vi "Coord window-PictureMap abs max.vi"(11 "Coordinates Listbox Item Names":string[][](array[string])) -> (1 "Auto-scale":bool, 3 "Absolute maximum coordinate (inc current position)":dbl)   [LabVIEW 2013]
panel:
  out "Absolute maximum coordinate in the list":dbl
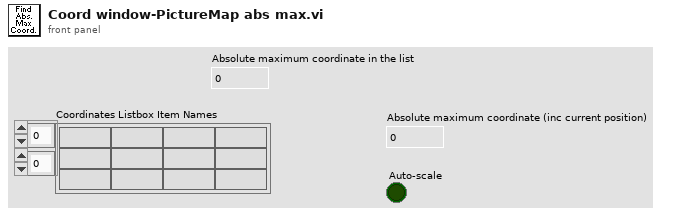
[diagram p1: front panel]
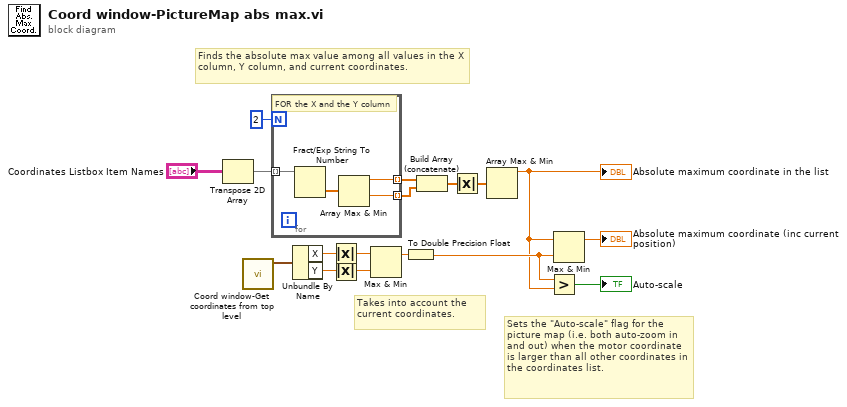
[diagram p0: block diagram]
diagram:
  # "Sets the \"Auto-scale\" flag for the picture map (i.e. both auto-zoom in and out) when the motor coordinate is larger than all other coordinates in the coordinates list."
  # "Takes into account the current coordinates."
  # "Finds the absolute max value among all values in the X column, Y column, and current coordinates."
  n1 = Transpose 2D Array(2D array="Coordinates Listbox Item Names") -> (transposed array=w13:string[][])
  n2 = call "Coord window-Get coordinates from top level.vi"() -> ("Coordinates"=w10:cluster{"X":sgl, "Y":sgl, "Z":sgl})  [unwired: 11 in]
  n3 = for {
    N: 2 -> [_]
    tunnel: w13 -> [w21] mode=indexing
    tunnel: [w19] -> w14 mode=indexing
    tunnel: [w18] -> w15 mode=indexing
    # "FOR the X and the Y column"
    n4 = Fract/Exp String To Number(string=w21) -> (number=w20:dbl[])  [unwired: 3 in, 1 out]
    n5 = Array Max & Min(array=w20) -> (max value=w19:dbl, min value=w18:dbl)  [unwired: 2 out]
  }
  n6 = Unbundle By Name(w10) -> ("X"=w9:sgl, "Y"=w8:sgl)
  n7 = Absolute Value(x=w9) -> (abs(x)=w7:sgl)
  n8 = Absolute Value(x=w8) -> (abs(x)=w6:sgl)
  n9 = Max & Min(x=w7, y=w6) -> (max(x,y)=w5:sgl)  [unwired: 1 out]
  n10 = To Double Precision Float(number=w5) -> (double precision float=w3:dbl)
  n11 = Build Array (concatenate)(w14, w15) -> (w16:dbl[])
  n12 = Absolute Value(x=w16) -> (abs(x)=w17:dbl[])
  n13 = Array Max & Min(array=w17) -> (max value=w2:dbl)  [unwired: 3 out]
  "Absolute maximum coordinate in the list" <- w2
  n14 = Greater?(x=w3, y=w2) -> (0:→"Auto-scale":bool)
  n15 = Max & Min(x=w2, y=w3) -> (max(x,y)=→"Absolute maximum coordinate (inc current position)":dbl)  [unwired: 1 out]
